vi "test_File or directory exists.vi"(8 "error in (no error)":errorcluster, 11 "TestCase in":refnum<class "[Test Case] File or directory exists.lvclass">) -> (0 "error out":errorcluster, 3 "TestCase out":refnum<class "[Test Case] File or directory exists.lvclass">)   [LabVIEW 2016, in "Tests.lvlib" / "[Test Case] File or directory exists.lvclass"]
uses:
  [Test Case] File or directory exists.lvclass
  [Test Case] File or directory exists.lvclass/[Test Case] File or directory exists.ctl
  classes/File Transfer Behavior/File Transfer Behavior.lvclass
  <vilib>/addons/_JKI Toolkits/VI Tester/TestCase.llb/TestCase.lvclass
  C:/Program Files (x86)/National Instruments/LabVIEW 2016/vi.lib/addons/_JKI Toolkits/VI Tester/TestCase.llb/TestCase.lvclass
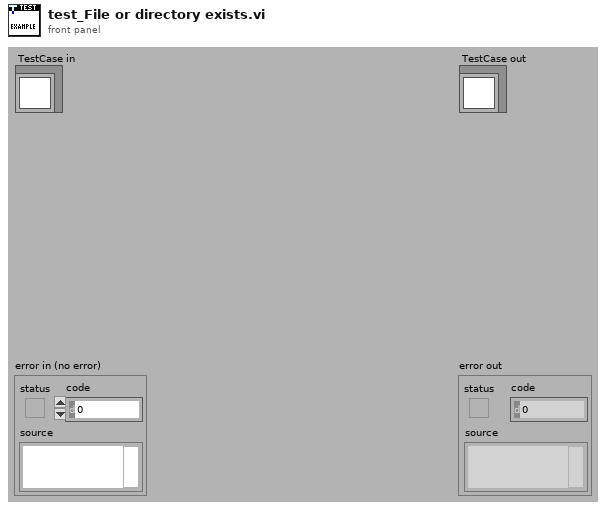
[diagram p1: front panel]
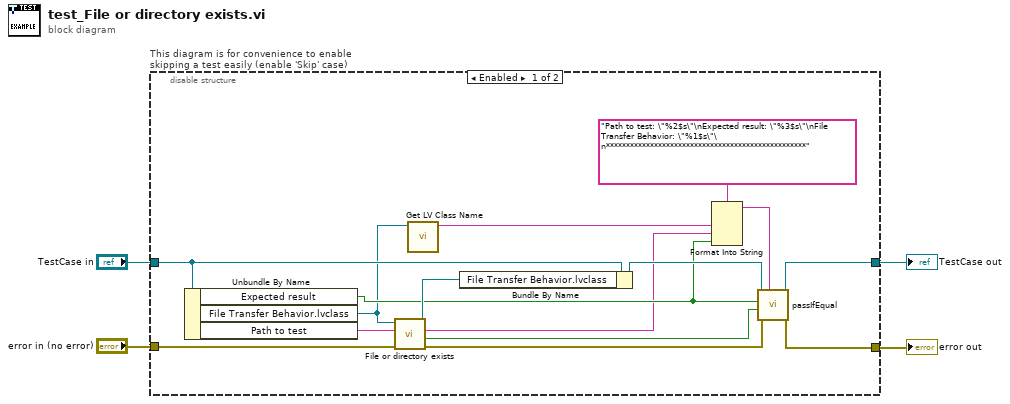
[diagram p0: block diagram]
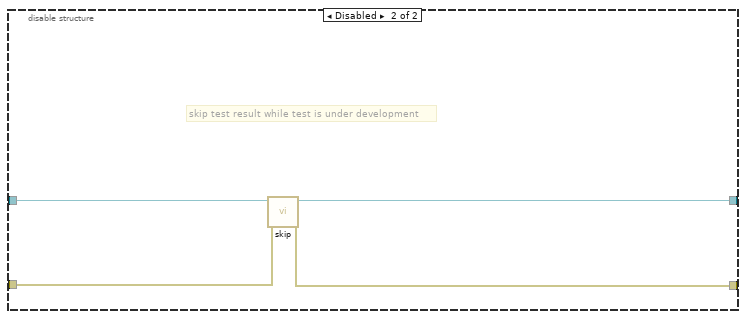
[diagram p2: hidden frame]
diagram:
  n1 = disable-structure "This diagram is for convenience to enable skipping a test easily (enable 'Skip' case)" shown="Enabled" {
    disable-tunnel: "TestCase in" -> [w13 w23]
    disable-tunnel: [w19 w21] -> w1
    disable-tunnel: [w18 w22] -> w3
    disable-tunnel: "error in (no error)" -> [w16 w20]
    frame Enabled {
      n2 = Unbundle By Name(w13) -> ("Expected result"=w8:bool, "File Transfer Behavior.lvclass"=w7:refnum<class "File Transfer Behavior.lvclass">, "Path to test"=w17:string)
      n3 = call-dynamic "File or directory exists.vi"("error in (no error)"=w16, "Path"=w17, "File Transfer Behavior in"=w7) -> ("error out"=w14:errorcluster, "Exists?"=w15:bool, "Path out (dup)"=w6:string, "File Transfer Behavior out"=w12:refnum<class "File Transfer Behavior.lvclass">)  [unwired: 4 in, 1 out]
      n4 = call <vilib>:"Get LV Class Name.vi"("object"=w7) -> ("class name"=w5:string)  [unwired: 9 in, 1 out]
      n5 = Bundle By Name(cluster=w13, "File Transfer Behavior.lvclass"=w12) -> (w11:refnum<class "[Test Case] File or directory exists.lvclass">)
      n6 = Format Into String(format string="Path to test: \"%2$s\"\nExpected result: \"%3$s\"\nFile Transfer Behavior: \"%1$s\"\n**************************************************", w5, w6, w8) -> (resulting string=w9:string)  [unwired: 2 in, 1 out]
      n7 = call-dynamic "passIfEqual.vi"("custom report message (\"\")"=w9, "error in (no error)"=w14, "y"=w15, "x"=w8, "TestCase in"=w11) -> ("error out"=w18:errorcluster, "TestCase out"=w19:refnum<class "[Test Case] File or directory exists.lvclass">)  [unwired: 5 in]
    }
    frame Disabled {
      # "skip test result while test is under development"
      n8 = call <vilib>:"skip.vi"("error in (no error)"=w20, "TestCase in"=w23) -> ("error out"=w22:errorcluster, "TestCase out"=w21:refnum<class "[Test Case] File or directory exists.lvclass">)  [unwired: 8 in]
    }
  }
  "error out" <- w3
  "TestCase out" <- w1
